vi "ParseEst.vi"(5 "String":string="*IDN?\n") -> (4 "Relé":bool, 6 "Sobrecalientamiento":bool, 8 "Remote":bool, 10 "Ajuste fino":bool, 14 "Bloqueado":bool, 15 "Mando Giratorio":bool)   [LabVIEW 2011]
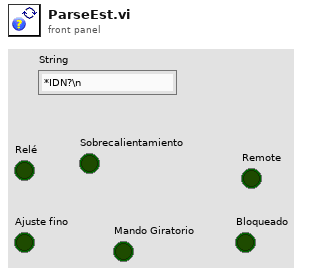
[diagram p1: front panel]
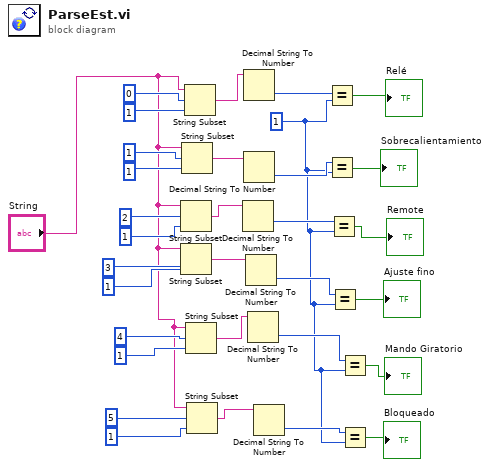
[diagram p0: block diagram]
diagram:
  w1 = 1
  n1 = String Subset(string="String", offset (0)=2, length (rest)=1) -> (substring=w9:string)
  n2 = String Subset(string="String", offset (0)=3, length (rest)=1) -> (substring=w10:string)
  n3 = String Subset(string="String", offset (0)=1, length (rest)=1) -> (substring=w8:string)
  n4 = String Subset(string="String", offset (0)=0, length (rest)=1) -> (substring=w19:string)
  n5 = String Subset(string="String", offset (0)=4, length (rest)=1) -> (substring=w11:string)
  n6 = String Subset(string="String", offset (0)=5, length (rest)=1) -> (substring=w12:string)
  n7 = Decimal String To Number(string=w9) -> (number=w5:i32)  [unwired: 2 in, 1 out]
  n8 = Decimal String To Number(string=w19) -> (number=w7:i32)  [unwired: 2 in, 1 out]
  n9 = Decimal String To Number(string=w8) -> (number=w6:i32)  [unwired: 2 in, 1 out]
  n10 = Decimal String To Number(string=w10) -> (number=w4:i32)  [unwired: 2 in, 1 out]
  n11 = Decimal String To Number(string=w11) -> (number=w3:i32)  [unwired: 2 in, 1 out]
  n12 = Decimal String To Number(string=w12) -> (number=w2:i32)  [unwired: 2 in, 1 out]
  n13 = Equal?(x=w7, y=w1) -> (x = y?=→"Relé":bool)
  n14 = Equal?(x=w6, y=w1) -> (x = y?=→"Sobrecalientamiento":bool)
  n15 = Equal?(x=w5, y=w1) -> (x = y?=→"Remote":bool)
  n16 = Equal?(x=w4, y=w1) -> (x = y?=→"Ajuste fino":bool)
  n17 = Equal?(x=w3, y=w1) -> (x = y?=→"Mando Giratorio":bool)
  n18 = Equal?(x=w2, y=w1) -> (x = y?=→"Bloqueado":bool)
